vi "Deploy.vi"() -> ()   [LabVIEW 2015]
uses:
  <vilib>/AppBuilder/AB_API_Simple/NI_App_Builder_API.lvlib
panel:
  out "error out":errorcluster
  in  "Stop":bool
  out "Control Value:Get All":cluster{"Name":string, "Variant Data":variant}[](array[cluster])
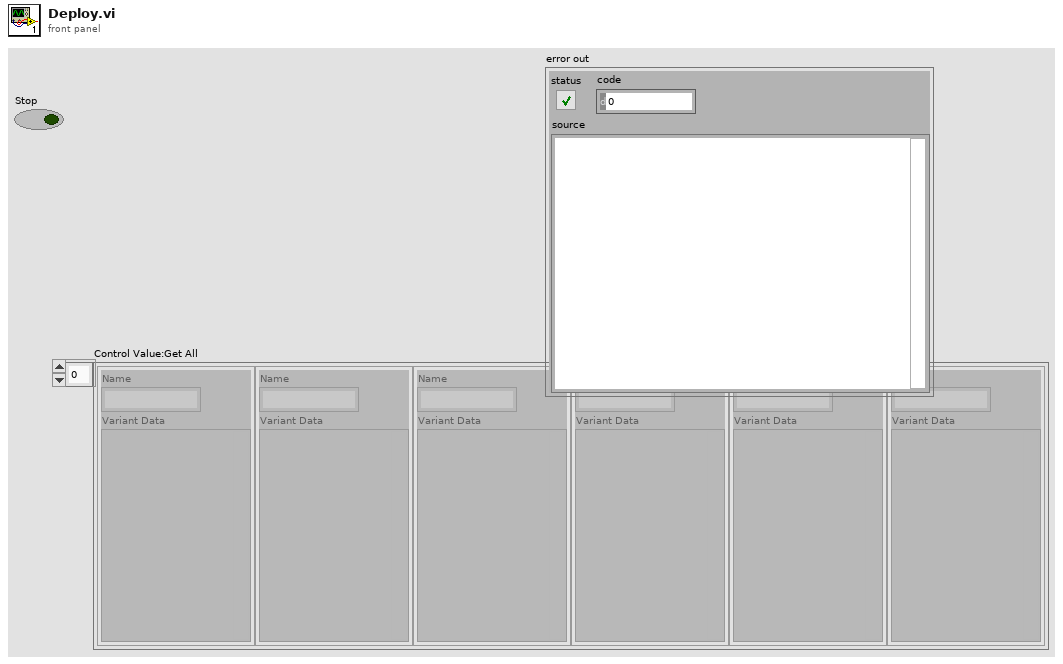
[diagram p1: front panel]
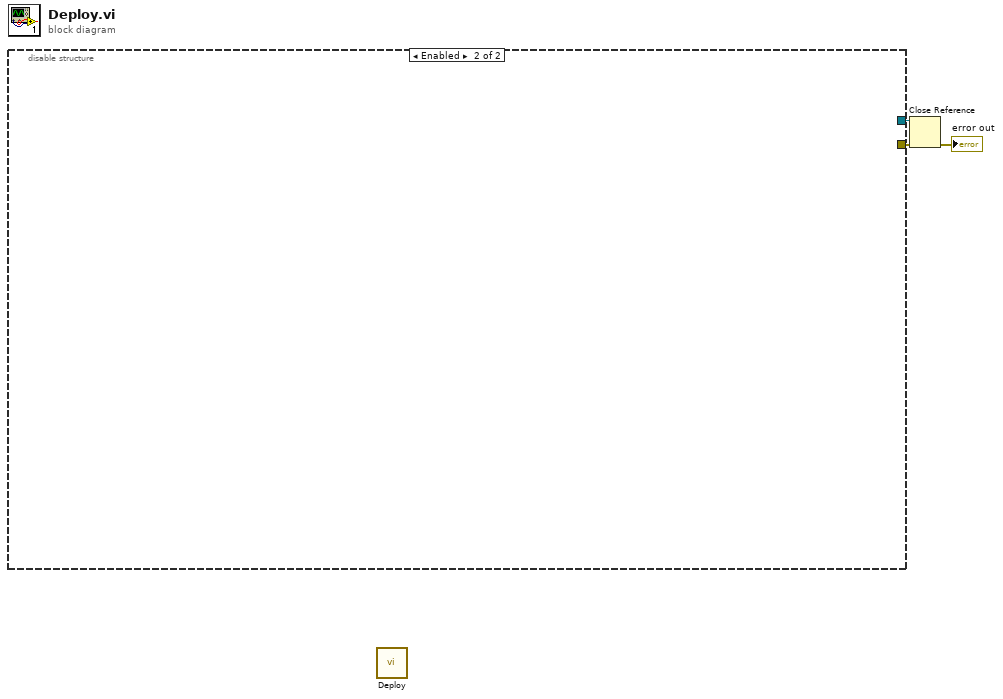
[diagram p0: block diagram]
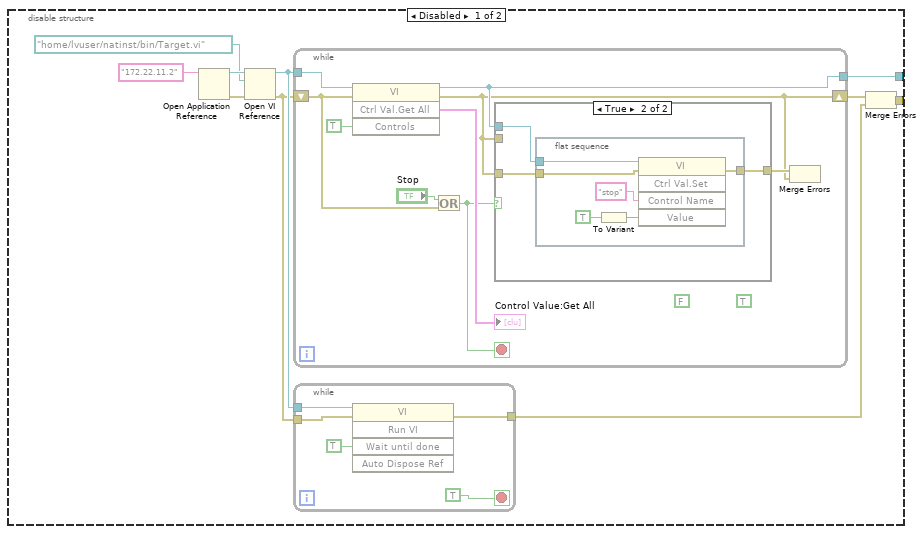
[diagram p2: hidden frame]
diagram:
  n1 = disable-structure shown="Enabled" {
    disable-tunnel: [w9 _] -> w3
    disable-tunnel: [w4 _] -> w2
    frame Disabled {
      n2 = Open Application Reference(11:"172.22.11.2" ("machine name (\"\":  open local reference)")) -> (0:w10:errorcluster, 3:w12:refnum<vi>)  [unwired: 3 in]
      n3 = Open VI Reference(application reference (local)=w12, vi path=path "/home/lvuser/natinst/bin/Target.vi", error in (no error)=w10) -> (vi reference=w8:refnum<vi>, error out=w6:errorcluster)  [unwired: 3 in]
      n4 = while {
        shift-right: [w20] -> w5
        shift-left: w6 -> [w27]
        tunnel: [w22] -> w9
        tunnel: w8 -> [w24]
        stop <- w19 stop-if-true
        (unwired) TRUE ("Wait Until Done")
        (unwired) FALSE ("Wait Until Done")
        n5 = invoke class="VI" method="Ctrl Val.Get All"(reference=w24, error in=w27, "Controls"=TRUE) -> (reference out=w22:refnum<vi>, error out=w20:errorcluster, "Get All Control Values Variant"=→"Control Value:Get All":cluster{"Name":string, "Variant Data":variant}[])  [unwired: 1 in, 1 out]
        n6 = Or(x="Stop", y=w27) -> (x .or. y?=w19:bool)
        n7 = case shown="True" w19 {
          tunnel: w22 -> [_ w31]
          tunnel: [w28 w30] -> w21
          tunnel: w20 -> [w28 _]
          tunnel: w20 -> [_ w29]
          frame False {
          }
          frame True {
            n8 = flat-sequence {
              tunnel: w31 -> [w36]
              tunnel: [w35] -> w30
              tunnel: w29 -> [w34]
              frame #0 {
                n9 = To Variant(anything=TRUE ("Stop")) -> (Variant=w33:variant)
                n10 = invoke class="VI" method="Ctrl Val.Set"(reference=w36, error in=w34, "Control Name"="stop", "Value"=w33) -> (error out=w35:errorcluster)  [unwired: 1 in, 4 out]
              }
            }
          }
        }
        n11 = Merge Errors(w21, w20) -> ()  [unwired: 1 out]
      }
      n12 = while {
        tunnel: w8 -> [w18]
        tunnel: [w16] -> w7
        tunnel: w6 -> [w15]
        stop <- TRUE stop-if-true
        n13 = invoke class="VI" method="Run VI"(reference=w18, error in=w15, "Wait until done"=TRUE ("Wait Until Done")) -> (error out=w16:errorcluster)  [unwired: 2 in, 4 out]
      }
      n14 = Merge Errors(w5, w7) -> (w4:errorcluster)
    }
    frame Enabled {
    }
  }
  n15 = call <vilib>:"Deploy.vi"() -> ()  [unwired: 11 in, 1 out]
  n16 = Close Reference(reference=w3, error in (no error)=w2) -> (error out=→"error out":errorcluster)
